vi "Indicator Init.vi"(7 "VolatusAPI":refnum<class "VolatusAPI.lvclass">, 8 "error in (no error)":errorcluster, 10 "JSON":string, 11 "Indicator in":refnum<class "Indicator.lvclass">) -> (0 "error out":errorcluster, 3 "Indicator out":refnum<class "Indicator.lvclass">)   [LabVIEW 2020, in "VolatusGUI.lvlib" / "Indicator.lvclass"]
uses:
  Indicator.lvclass
  Indicator.lvclass/Indicator.ctl
  Volatus/VolatusAPI/VolatusAPI.lvclass
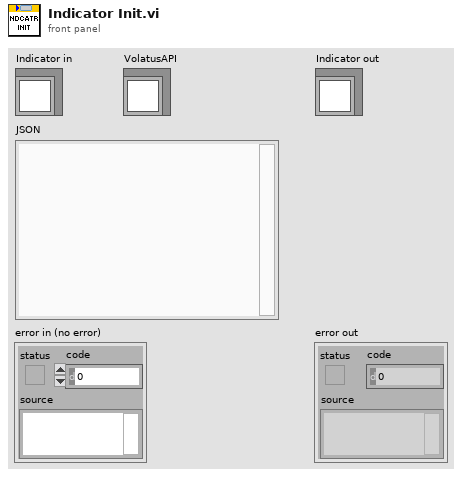
[diagram p1: front panel]
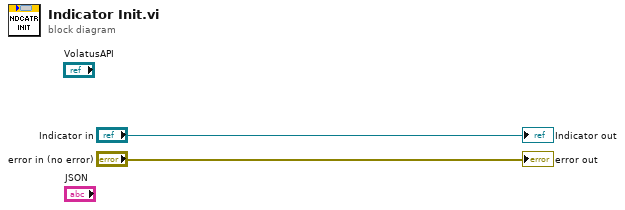
[diagram p0: block diagram]
diagram:
  "error out" <- "error in (no error)"
  "Indicator out" <- "Indicator in"
